vi "电机定位.vi"(4 "细分设置":dbl=8.0, 6 "电机急停":bool, 7 "等待时间(ms)":u32=40, 8 "精度":dbl=0.001, 9 "X":dbl, 11 "VISA I":refnum<visa-resource-name>) -> (0 "Y":dbl, 1 "X":dbl, 3 "VISA O":refnum<visa-resource-name>)   [LabVIEW 2016]
panel:
  in  "Y":dbl
  in  "确定":bool
  in  "ESC":bool
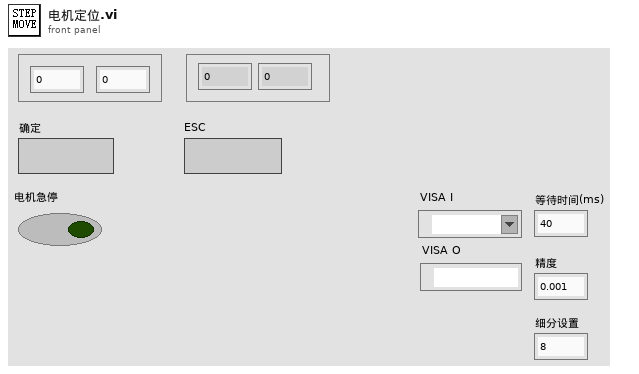
[diagram p1: front panel]
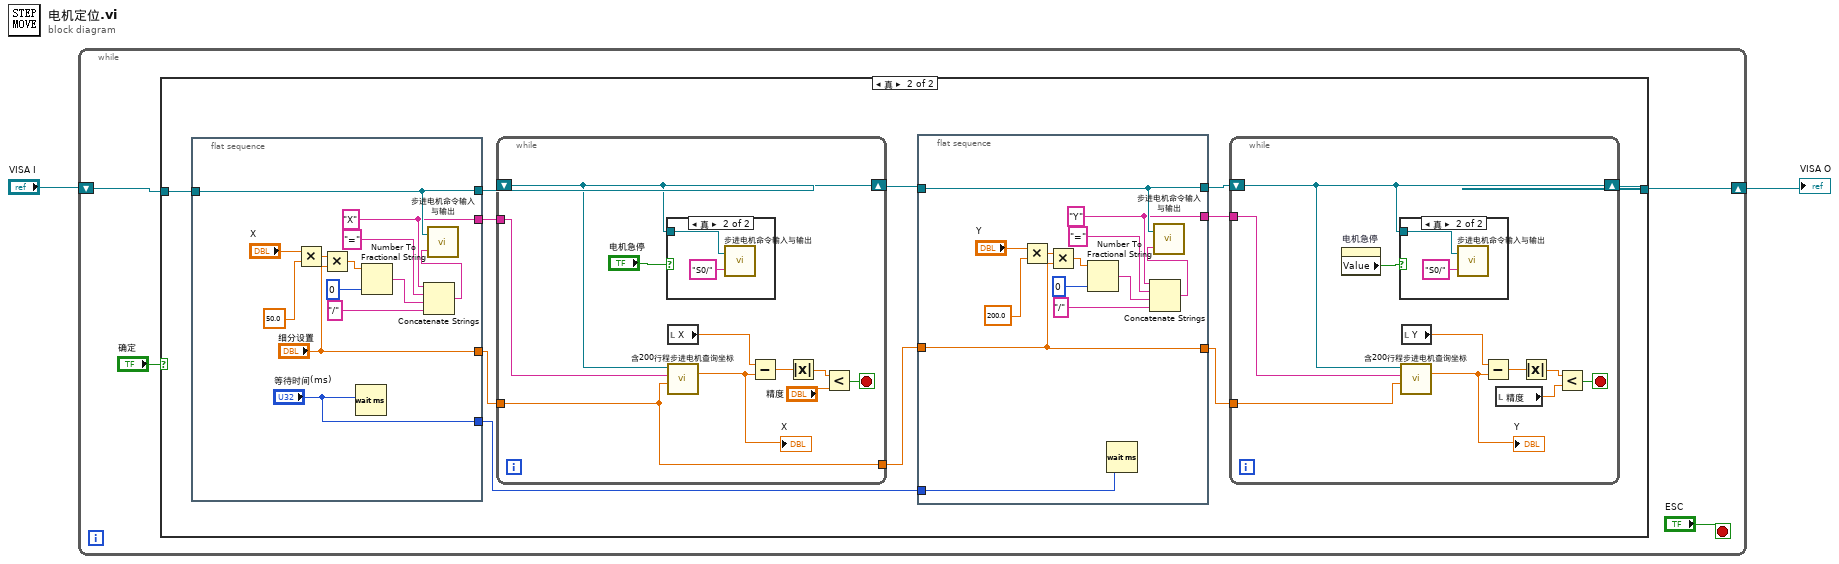
[diagram p0: block diagram]
diagram:
  n1 = while {
    shift-right: [w5] -> w2
    shift-left: "VISA I" -> [w6]
    stop <- "ESC" stop-if-true
    n2 = case shown="真" "确定" {
      tunnel: w6 -> [w7 w17]
      tunnel: [w7 w10] -> w5
      frame False {
      }
      frame True {
        n3 = flat-sequence {
          tunnel: w17 -> [w60]
          tunnel: [w60] -> w18
          tunnel: ["细分设置"] -> w16
          tunnel: [w57] -> w15
          tunnel: ["等待时间(ms)"] -> w9
          frame #0 {
            w57 = "X"
            n4 = Multiply(x="X", y=50.0 ("x")) -> (x*y=w63:dbl)
            n5 = Multiply(x=w63, y="细分设置") -> (x*y=w68:dbl)
            n6 = Wait (ms)(milliseconds to wait="等待时间(ms)") -> ()  [unwired: 1 out]
            n7 = Number To Fractional String(number=w68, precision (6)=i16 0 ("精度(6)")) -> (F-format string=w66:string)  [unwired: 2 out]
            n8 = Concatenate Strings(w57, "=" ("字符串"), w66, "/" ("字符串")) -> (w62:string)
            n9 = call "步进电机命令输入与输出.vi"("输入字符串"=w62, "串口通信端口"=w60) -> ()  [unwired: 1 out]
          }
        }
        n10 = while {
          tunnel: w16 -> [w45]
          tunnel: w15 -> [w46]
          tunnel: [w45] -> w8
          shift-right: [w50] -> w11
          shift-left: w18 -> [w50]
          stop <- w53 stop-if-true
          n11 = case shown="真" "电机急停" {
            tunnel: w50 -> [_ w54]
            frame False {
            }
            frame True {
              n12 = call "步进电机命令输入与输出.vi"("输入字符串"="S0/", "串口通信端口"=w54) -> ()  [unwired: 1 out]
            }
          }
          n13 = local read "X"() -> (w48:dbl)
          n14 = call "含200行程步进电机查询坐标.vi"("细分设置"=w45, "查询坐标轴"=w46, "串口通信端口"=w50) -> ("坐标(mm)"=w47:dbl)  [unwired: 8 in]
          "X" <- w47
          n15 = Subtract(x=w48, y=w47) -> (x-y=w52:dbl)
          n16 = Absolute Value(x=w52) -> (abs(x)=w51:dbl)
          n17 = Less?(x=w51, y="精度") -> (x < y?=w53:bool)
        }
        n18 = flat-sequence {
          tunnel: w11 -> [w35]
          tunnel: [w35] -> w14
          tunnel: [w31] -> w13
          tunnel: [w33] -> w12
          tunnel: w9 -> [w32]
          tunnel: w8 -> [w31]
          frame #0 {
            w33 = "Y"
            n19 = Multiply(x="Y", y=200.0 ("x")) -> (x*y=w38:dbl)
            n20 = Multiply(x=w38, y=w31) -> (x*y=w43:dbl)
            n21 = Number To Fractional String(number=w43, precision (6)=i16 0 ("精度(6)")) -> (F-format string=w41:string)  [unwired: 2 out]
            n22 = Wait (ms)(milliseconds to wait=w32) -> ()  [unwired: 1 out]
            n23 = Concatenate Strings(w33, "=" ("字符串"), w41, "/" ("字符串")) -> (w37:string)
            n24 = call "步进电机命令输入与输出.vi"("输入字符串"=w37, "串口通信端口"=w35) -> ()  [unwired: 1 out]
          }
        }
        n25 = while {
          tunnel: w13 -> [w22]
          tunnel: w12 -> [w21]
          shift-right: [w25] -> w10
          shift-left: w14 -> [w25]
          stop <- w28 stop-if-true
          n26 = property on="电机急停" class="Bool (严格)"() -> ("Value"=w19:bool)  [unwired: 2 in, 2 out]
          n27 = case shown="真" w19 {
            tunnel: w25 -> [_ w29]
            frame False {
            }
            frame True {
              n28 = call "步进电机命令输入与输出.vi"("输入字符串"="S0/", "串口通信端口"=w29) -> ()  [unwired: 1 out]
            }
          }
          n29 = call "含200行程步进电机查询坐标.vi"("细分设置"=w22, "查询坐标轴"=w21, "串口通信端口"=w25) -> ("坐标(mm)"=w23:dbl)  [unwired: 8 in]
          "Y" <- w23
          n30 = local read "Y"() -> (w24:dbl)
          n31 = Subtract(x=w24, y=w23) -> (x-y=w27:dbl)
          n32 = local read "精度"() -> (w20:dbl)
          n33 = Absolute Value(x=w27) -> (abs(x)=w26:dbl)
          n34 = Less?(x=w26, y=w20) -> (x < y?=w28:bool)
        }
      }
    }
  }
  "VISA O" <- w2
